vi "set_multiramp_soak_configuration.vi"(8 "error in (no error)":errorcluster, 10 "Configuration":string(combo)="0", 11 "connection ID":refnum<k5>) -> (0 "error out":errorcluster, 3 "connection ID out":refnum<k5>)   [LabVIEW 2018]
panel:
  out "bytes written":i32
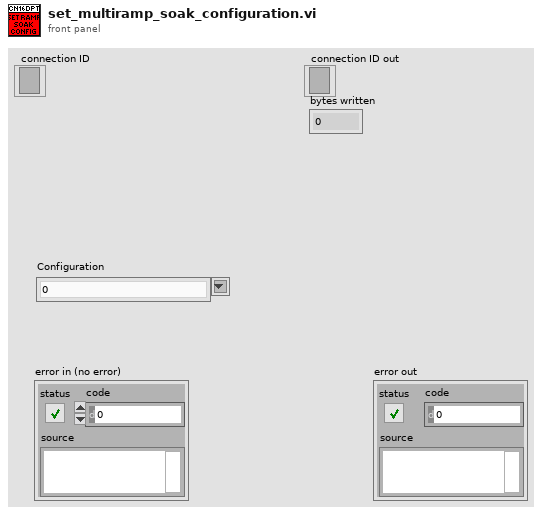
[diagram p1: front panel]
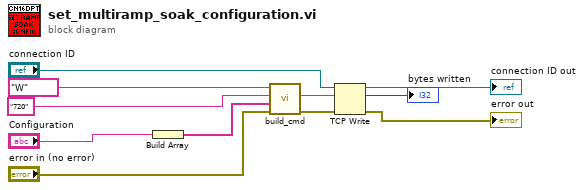
[diagram p0: block diagram]
diagram:
  n1 = Build Array("Configuration") -> (w4:string[])
  n2 = call "build_cmd.vi"("error in (no error)"="error in (no error)", "Parameter list"=w4, "Command ID"="720", "Command class"="W") -> ("error out"=w8:errorcluster, "Command"=w7:string)  [unwired: 6 in]
  n3 = TCP Write(connection ID="connection ID", data in=w7, error in (no error)=w8) -> (connection ID out=→"connection ID out":refnum<k5>, bytes written=→"bytes written":i32, error out=→"error out":errorcluster)  [unwired: 1 in]
